vi "test_StartSMO.vi"(8 "error in (no error)":errorcluster, 11 "TestCase in":refnum<class "SMO_TestCase.lvclass">) -> (0 "error out":errorcluster, 3 "TestCase out":refnum<class "SMO_TestCase.lvclass">)   [LabVIEW 2013, in "SMO_TestCase.lvclass"]
uses:
  SMO_TestCase.lvclass
  SMO_TestCase.lvclass/SMO_TestCase.ctl
  <vilib>/addons/_JKI Toolkits/VI Tester/TestCase.llb/TestCase.lvclass
  src/SMO/SMO.lvclass
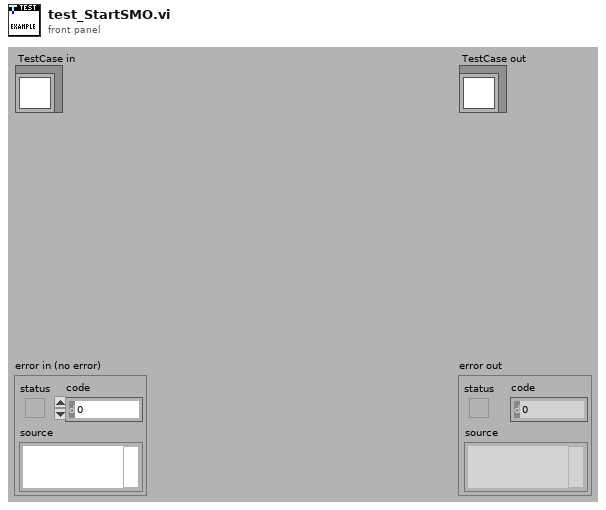
[diagram p1: front panel]
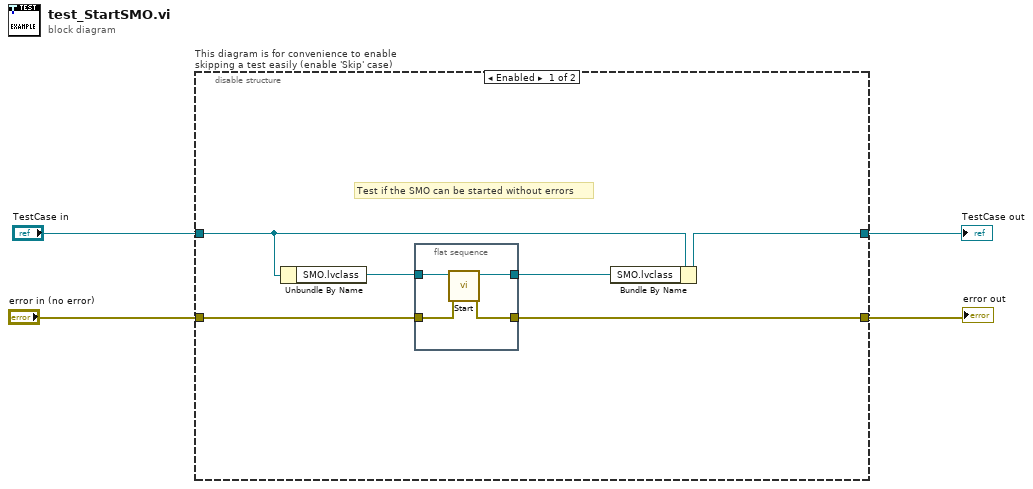
[diagram p0: block diagram]
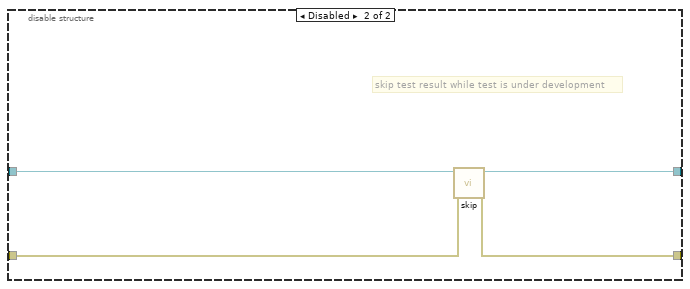
[diagram p2: hidden frame]
diagram:
  n1 = disable-structure "This diagram is for convenience to enable skipping a test easily (enable 'Skip' case)" shown="Enabled" {
    disable-tunnel: "TestCase in" -> [w7 w18]
    disable-tunnel: [w6 w16] -> w1
    disable-tunnel: [w8 w17] -> w3
    disable-tunnel: "error in (no error)" -> [w9 w15]
    frame Enabled {
      # "Test if the SMO can be started without errors"
      n2 = Unbundle By Name(w7) -> ("SMO.lvclass"=w10:refnum<class "SMO.lvclass">)
      n3 = flat-sequence {
        tunnel: w10 -> [w14]
        tunnel: w9 -> [w13]
        tunnel: [w12] -> w8
        tunnel: [w11] -> w5
        frame #0 {
          n4 = call "Start.vi"("error in (no error)"=w13, "SMO"=w14) -> ("error out"=w12:errorcluster, "SMO out"=w11:refnum<class "SMO.lvclass">)  [unwired: 8 in]
        }
      }
      n5 = Bundle By Name(cluster=w7, "SMO.lvclass"=w5) -> (w6:refnum<class "SMO_TestCase.lvclass">)
    }
    frame Disabled {
      # "skip test result while test is under development"
      n6 = call <vilib>:"skip.vi"("error in (no error)"=w15, "TestCase in"=w18) -> ("error out"=w17:errorcluster, "TestCase out"=w16:refnum<class "SMO_TestCase.lvclass">)  [unwired: 8 in]
    }
  }
  "error out" <- w3
  "TestCase out" <- w1
